vi "+S2C_M2p5942_Process.vi"(8 "Error In":errorcluster) -> (0 "Error Out":errorcluster)   [LabVIEW 2024]
uses:
  VIs/S2C_M2p5942_Proc_Globals.vi
panel:
  out "Err":bool
  in  "Clear":bool
  out "Exit":bool
  in  "LogDepth":u32=10 caption="Log Depth"
  in  "CtrlTab":T1(tab)
  in  "P1":T2={"Initialize"={"Index"=0, "IP Address"="<Not Used>", "Device"=0, "P1C1Exe"=FALSE}, "DeviceInfo"={"Device Name"="", "Serial Number"="", "Memory (MB)"="", "ClearExe"=FALSE}} {"Initialize"."Device" items=["Card", "digitizerNETBOX"]}
  in  "P2":T3={"Channels"={"CH1"={"CH0 Enable"=TRUE, "CH0 Range"=2, "CH0 Term"=0, "CH0 Type"=0, "CH0 Offset"=0}, "CH2"={"CH1 Enable"=TRUE, "CH1 Range"=2, "CH1 Term"=0, "CH1 Type"=0, "CH1 Offset"=0}, "CH3"={"CH2 Enable"=TRUE, "CH2 Range"=2, "CH2 Term"=0, "CH2 Type"=0, "CH2 Offset"=0}, "CH4"={"CH3 Enable"=TRUE, "CH3 Range"=2, "CH3 Term"=0, "CH3 Type"=0, "CH3 Offset"=0}, "P2C1Exe"=FALSE}, "Mode Settings"={"Mode"=0, "Memory"=16384, "Segment Size"=1024, "PostTrigger"=8192, "PreTrigger"=32, "ABA Mode"=16, "P2C2Exe"=FALSE}} {"Mode Settings"."ABA Mode" min=2 max=65535 step=1; "Mode Settings"."PostTrigger" min=4 step=4; "Mode Settings"."PreTrigger" min=4 max=8176 step=4; "Mode Settings"."Segment Size" min=8 step=4; "Mode Settings"."Memory" min=8 step=4; "Mode Settings"."Mode" items=["Singleshot", "Multiple Recording", "Gated Sampling", "ABA Mode"]; "Channels"."CH4"."CH3 Type" items=["Single-ended", "Differential"]; "Channels"."CH4"."CH3 Term" items=["1 MOhm", "50 Ohm"]; "Channels"."CH4"."CH3 Range" items=["±200 mV", "±500 mV", "±1000 mV", "±2000 mV", "±5000 mV", "±10000 mV"]; "Channels"."CH3"."CH2 Type" items=["Single-ended", "Differential"]; "Channels"."CH3"."CH2 Term" items=["1 MOhm", "50 Ohm"]; "Channels"."CH3"."CH2 Range" items=["±200 mV", "±500 mV", "±1000 mV", "±2000 mV", "±5000 mV", "±10000 mV"]; "Channels"."CH2"."CH1 Type" items=["Single-ended", "Differential"]; "Channels"."CH2"."CH1 Term" items=["1 MOhm", "50 Ohm"]; "Channels"."CH2"."CH1 Range" items=["±200 mV", "±500 mV", "±1000 mV", "±2000 mV", "±5000 mV", "±10000 mV"]; "Channels"."CH1"."CH0 Type" items=["Single-ended", "Differential"]; "Channels"."CH1"."CH0 Term" items=["1 MOhm", "50 Ohm"]; "Channels"."CH1"."CH0 Range" items=["±200 mV", "±500 mV", "±1000 mV", "±2000 mV", "±5000 mV", "±10000 mV"]}
  in  "P3":T4={"Trigger Settings"={"Trigger Source"=0, "External Trigger"=0, "EXT Trig Level 0"=1500, "EXT Trig Term"=TRUE, "Channel Trigger"=0, "CH Trig Level 0"=0, "CH Trig Level 1"=0, "Trigger Delay"=0, "P3C1Exe"=FALSE}, "Clock Settings"={"Clock Mode"=0, "Sampling Rate (kHz)"=10000.0, "Clock Output"=TRUE, "Termination"=TRUE, "Ref. Clock (MHz)"=10.0, "Threshold (mV)"=1500, "P3C2Exe"=FALSE}} {"Clock Settings"."Threshold (mV)" min=-5000 max=5000; "Clock Settings"."Sampling Rate (kHz)" min=1.0 max=5000000.0; "Clock Settings"."Ref. Clock (MHz)" min=0.0 max=125000.0; "Clock Settings"."Clock Mode" items=["Internal Clock Quartz", "External Clock", "External Reference Clock"]; "Trigger Settings"."Trigger Delay" max=65535 step=1; "Trigger Settings"."External Trigger" items=["None", "Pos. Edge", "Neg. Edge", "Any Edge", "High Level", "Low Level"]; "Trigger Settings"."Channel Trigger" items=["None", "Pos. Edge", "Neg. Edge", "Any Edge", "Pos. Rearm", "Neg. Rearm", "Enter Window", "Leave Window", "In Win", "Out Win"]; "Trigger Settings"."Trigger Source" items=["Software Trigger", "External Trigger", "Channel 0 Trigger", "Channel 1 Trigger", "Channel 2 Trigger", "Channel 3 Trigger", "Channel 4 Trigger", "Channel 5 Trigger", "Channel 6 Trigger", "Channel 7 Trigger"]}
  in  "P4":T5 {"Multi Purpose IO"."X3 Trigger Mode" items=["Pos. Edge", "Neg. Edge", "Any Edge", "High Level", "Low Level", "PW Long Pos.", "PW Long Neg.", "PW Short Pos.", "PW Short Neg."]; "Multi Purpose IO"."X2 Trigger Mode" items=["Pos. Edge", "Neg. Edge", "Any Edge", "High Level", "Low Level", "PW Long Pos.", "PW Long Neg.", "PW Short Pos.", "PW Short Neg."]; "Multi Purpose IO"."X1 Trigger Mode" items=["Pos. Edge", "Neg. Edge", "Any Edge", "High Level", "Low Level", "PW Long Pos.", "PW Long Neg.", "PW Short Pos.", "PW Short Neg."]; "Multi Purpose IO"."X3 Mode" items=["Disable", "Asynchronous Out", "Asynchronous In", "Trigger Out", "Trigger In", "Clock Out", "Digital In", "Show Run State", "Show Arm State", "Show Sync Arm State"]; "Multi Purpose IO"."X2 Mode" items=["Disable", "Asynchronous Out", "Asynchronous In", "Trigger Out", "Trigger In", "Clock Out", "Digital In", "Show Run State", "Show Arm State", "Show Sync Arm State"]; "Multi Purpose IO"."X1 Mode" items=["Disable", "Asynchronous Out", "Asynchronous In", "Trigger Out", "Trigger In", "Clock Out", "Digital In", "Show Run State", "Show Arm State", "Show Sync Arm State"]; "Multi Purpose IO"."X0 Mode" items=["Disable", "Asynchronous Out", "Trigger Out", "Clock Out", "Show Run State", "Show Arm State", "Show Sync Arm State"]}
  in  "P5":T6={"Acquisition"={"Single Shot"=FALSE, "Loop"=FALSE, "Force Trigger"=FALSE, "Status"="<Status>", "Stop"=FALSE, "Graph"=[]}}
  in  "CommLog":string caption="Communication Log"
  # "Main Cluster:\n394x886\n1 = 355x876\n2 = 355x438\n3 = 355x292\n4 = 163x438\n6 = 163x292\n8 = 163x219 \n\nSubTab 369x886\nSubClust 359x876"
  # "M2p5942 Driver Panel"
  # "Range"
  # "Term"
  # "Type"
  # "Offset"
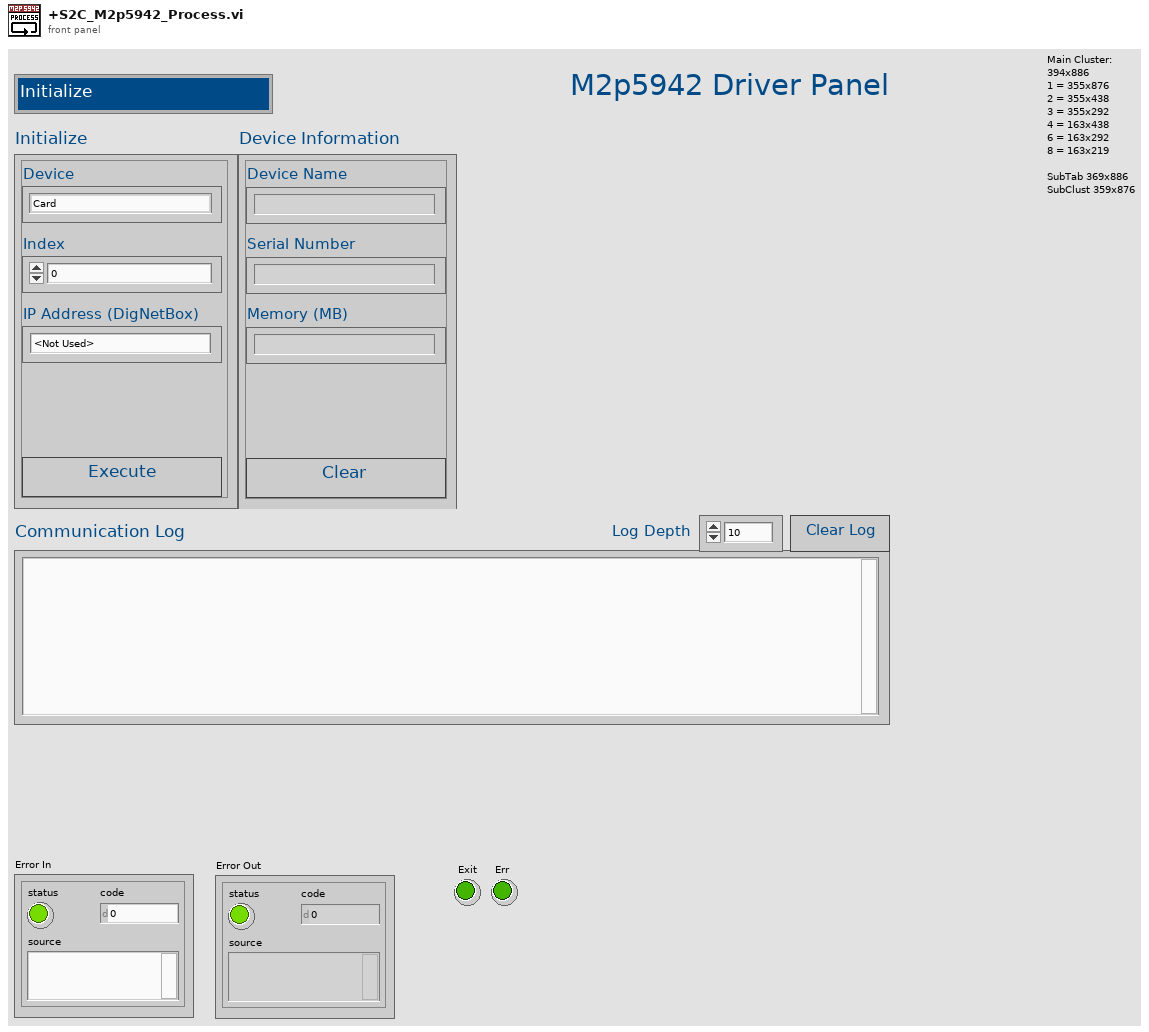
[diagram p1: front panel]
types:
  T1 = enum32{"Initialize", "Channels", "Trigger", "Multi Purpose IO", "Acquisition"}
  T2 = cluster{"Initialize":cluster{"Index":u32, "IP Address":string, "Device":u16, "P1C1Exe":bool}, "DeviceInfo":cluster{"Device Name":string, "Serial Number":string, "Memory (MB)":string, "ClearExe":bool}}
  T3 = cluster{"Channels":cluster{"CH1":cluster{"CH0 Enable":bool, "CH0 Range":u16, "CH0 Term":u16, "CH0 Type":u16, "CH0 Offset":i32}, "CH2":cluster{"CH1 Enable":bool, "CH1 Range":u16, "CH1 Term":u16, "CH1 Type":u16, "CH1 Offset":i32}, "CH3":cluster{"CH2 Enable":bool, "CH2 Range":u16, "CH2 Term":u16, "CH2 Type":u16, "CH2 Offset":i32}, "CH4":cluster{"CH3 Enable":bool, "CH3 Range":u16, "CH3 Term":u16, "CH3 Type":u16, "CH3 Offset":i32}, "P2C1Exe":bool}, "Mode Settings":cluster{"Mode":u16, "Memory":u32, "Segment Size":u32, "PostTrigger":u32, "PreTrigger":u32, "ABA Mode":u32, "P2C2Exe":bool}}
  T4 = cluster{"Trigger Settings":cluster{"Trigger Source":u16, "External Trigger":u16, "EXT Trig Level 0":i32, "EXT Trig Term":bool, "Channel Trigger":u16, "CH Trig Level 0":i32, "CH Trig Level 1":i32, "Trigger Delay":u32, "P3C1Exe":bool}, "Clock Settings":cluster{"Clock Mode":u16, "Sampling Rate (kHz)":dbl, "Clock Output":bool, "Termination":bool, "Ref. Clock (MHz)":dbl, "Threshold (mV)":i32, "P3C2Exe":bool}}
  T5 = cluster{"Multi Purpose IO":cluster{"X0 Mode":u16, "X1 Mode":u16, "X2 Mode":u16, "X3 Mode":u16, "X0 Send":bool, "X1 Send":bool, "X2 Send":bool, "X3 Send":bool, "X1 Trigger Mode":u16, "X2 Trigger Mode":u16, "X3 Trigger Mode":u16, "X1 Pulsewidth":u32, "X2 Pulsewidth":u32, "X3 Pulsewidth":u32, "ASync Read":bool, "ASync Data":i32}}
  T6 = cluster{"Acquisition":cluster{"Single Shot":bool, "Loop":bool, "Force Trigger":bool, "Status":string, "Stop":bool, "Graph":sgl[][]}}
  T7 = cluster{"Device Name":string, "Serial Number":string, "Memory (MB)":string, "ClearExe":bool}
  T8 = cluster{"Caller-Q":refnum<queue>, "Command":string, "Return":string, "Data":variant, "Timeout":dbl}
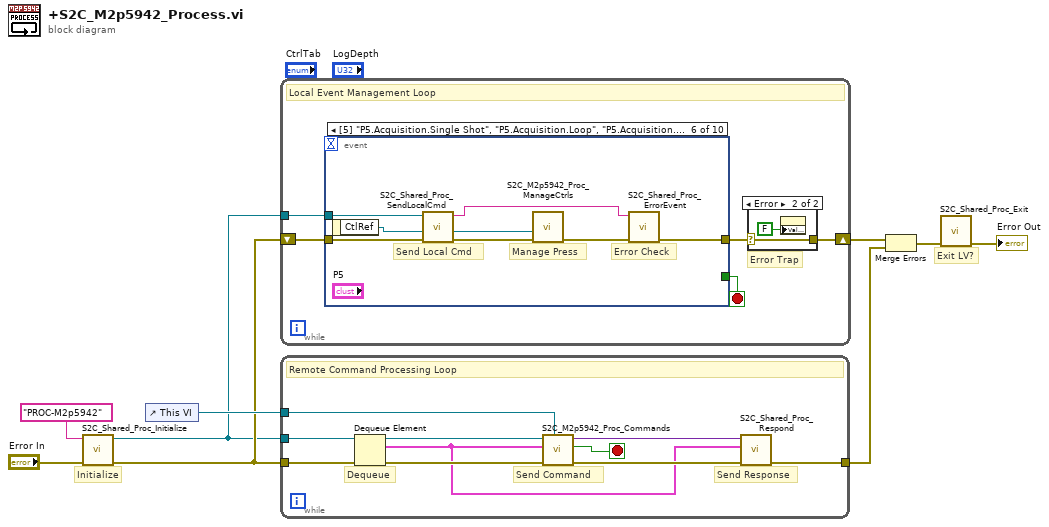
[diagram p0: block diagram]
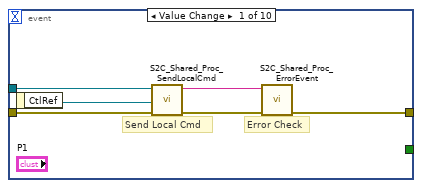
[diagram p3: hidden frame]
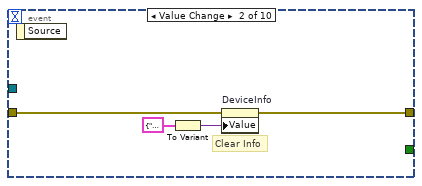
[diagram p4: hidden frame]
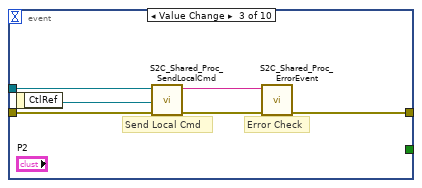
[diagram p5: hidden frame]
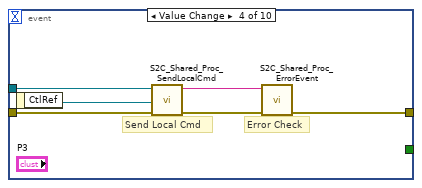
[diagram p6: hidden frame]
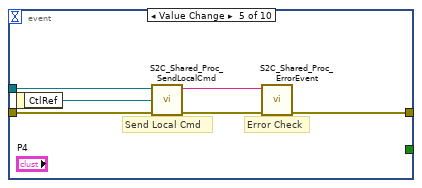
[diagram p7: hidden frame]
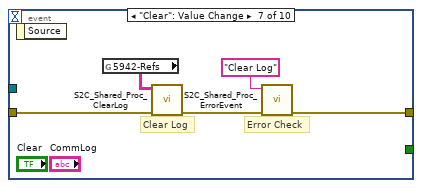
[diagram p8: hidden frame]
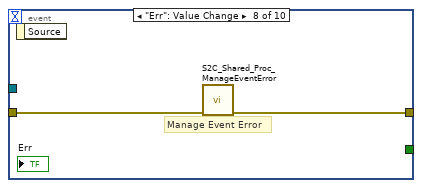
[diagram p9: hidden frame]
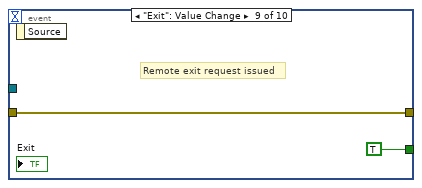
[diagram p10: hidden frame]
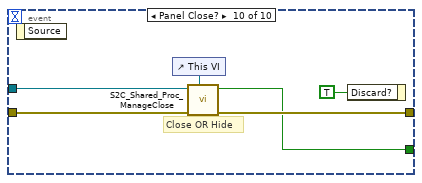
[diagram p11: hidden frame]
diagram:
  # "Exit LV?"
  # "Initialize"
  n1 = call "S2C_Shared_Proc_Initialize.vi"("Error In"="Error In", "Q-Name"="PROC-M2p5942" ("name (unnamed)")) -> ("Error Out"=w4:errorcluster, "Q-Ref"=w1:refnum<queue>)  [unwired: 8 in]
  n2 = control-ref of="This VI"() -> (w5:refnum<vi>)
  n3 = while {
    tunnel: w1 -> [w12]
    shift-right: [w10] -> w7
    shift-left: w4 -> [w14]
    stop <- w13 stop-if-true
    # "Error Trap"
    # "Local Event Management Loop"
    n4 = event shown="[5] \"P5.Acquisition.Single Shot\", \"P5.Acquisition.Loop\", \"P5.Acquisition.Stop\": Value Change" {
      selector: _ -> [_ _ _ _ _ _ _ _ _ _]
      dyn-events: _ -> [_ _ _ _ _ _ _ _ _ _]
      timeout: _ -> [_ _ _ _ _ _ _ _ _ _]
      tunnel: w14 -> [w23 w27 w33 w39 w43 w51 w57 w59 w61 w66]
      tunnel: w12 -> [w21 _ w31 w37 w41 w50 _ _ _ w64]
      tunnel: [w20 w26 w30 w36 w40 w49 w55 w58 w61 w65] -> w11
      tunnel: [_ _ _ _ _ _ _ _ TRUE ("Discard?") w63] -> w13
      event "P1.Initialize.P1C1Exe": Value Change {
        # "Error Check"
        # "Send Local Cmd"
        n5 = event-data() -> ("CtlRef"=w22:refnum<vi>)  [unwired: 1 in]
        n6 = call "S2C_Shared_Proc_SendLocalCmd.vi"("Error In"=w23, "ExeRef"=w22, "Q-Ref"=w21) -> ("Error Out"=w19:errorcluster, "Command"=w18:string)  [unwired: 7 in]
        n7 = call "S2C_Shared_Proc_ErrorEvent.vi"("Error In"=w19, "Command"=w18) -> ("Error Out"=w20:errorcluster)  [unwired: 9 in]
      }
      event "P1.DeviceInfo.ClearExe": Value Change {
        # "Clear Info"
        n8 = event-data() -> ()  [unwired: 1 in, 1 out]
        n9 = To Variant(anything=T7 {"Device Name"="", "Serial Number"="", "Memory (MB)"="", "ClearExe"=FALSE} ("DeviceInfo")) -> (Variant=w25:variant)
        n10 = property on="DeviceInfo" class="Clust"(error in=w27, "Value"=w25) -> (error out=w26:errorcluster)  [unwired: 1 in, 1 out]
      }
      event "P2.Channels.P2C1Exe", "P2.Mode Settings.P2C2Exe": Value Change {
        # "Error Check"
        # "Send Local Cmd"
        n11 = event-data() -> ("CtlRef"=w32:refnum<vi>)  [unwired: 1 in]
        n12 = call "S2C_Shared_Proc_SendLocalCmd.vi"("Error In"=w33, "ExeRef"=w32, "Q-Ref"=w31) -> ("Error Out"=w29:errorcluster, "Command"=w28:string)  [unwired: 7 in]
        n13 = call "S2C_Shared_Proc_ErrorEvent.vi"("Error In"=w29, "Command"=w28) -> ("Error Out"=w30:errorcluster)  [unwired: 9 in]
      }
      event "P3.Trigger Settings.P3C1Exe", "P3.Clock Settings.P3C2Exe": Value Change {
        # "Error Check"
        # "Send Local Cmd"
        n14 = event-data() -> ("CtlRef"=w38:refnum<vi>)  [unwired: 1 in]
        n15 = call "S2C_Shared_Proc_SendLocalCmd.vi"("Error In"=w39, "ExeRef"=w38, "Q-Ref"=w37) -> ("Error Out"=w35:errorcluster, "Command"=w34:string)  [unwired: 7 in]
        n16 = call "S2C_Shared_Proc_ErrorEvent.vi"("Error In"=w35, "Command"=w34) -> ("Error Out"=w36:errorcluster)  [unwired: 9 in]
      }
      event "P4.Multi Purpose IO.X0 Send", "P4.Multi Purpose IO.X1 Send", "P4.Multi Purpose IO.X2 Send", "P4.Multi Purpose IO.X3 Send", "P4.Multi Purpose IO.ASync Read": Value Change {
        # "Error Check"
        # "Send Local Cmd"
        n17 = event-data() -> ("CtlRef"=w42:refnum<vi>)  [unwired: 1 in]
        n18 = call "S2C_Shared_Proc_SendLocalCmd.vi"("Error In"=w43, "ExeRef"=w42, "Q-Ref"=w41) -> ("Error Out"=w45:errorcluster, "Command"=w44:string)  [unwired: 7 in]
        n19 = call "S2C_Shared_Proc_ErrorEvent.vi"("Error In"=w45, "Command"=w44) -> ("Error Out"=w40:errorcluster)  [unwired: 9 in]
      }
      event "P5.Acquisition.Single Shot", "P5.Acquisition.Loop", "P5.Acquisition.Stop": Value Change {
        # "Manage Press"
        # "Error Check"
        # "Send Local Cmd"
        n20 = event-data() -> ("CtlRef"=w46:refnum<vi>)  [unwired: 1 in]
        n21 = call "S2C_Shared_Proc_SendLocalCmd.vi"("Error In"=w51, "ExeRef"=w46, "Q-Ref"=w50) -> ("Error Out"=w48:errorcluster, "Command"=w52:string)  [unwired: 7 in]
        n22 = call "S2C_M2p5942_Proc_ManageCtrls.vi"("Error In"=w48, "CtlRef"=w46) -> ("Error Out"=w47:errorcluster)  [unwired: 9 in]
        n23 = call "S2C_Shared_Proc_ErrorEvent.vi"("Error In"=w47, "Command"=w52) -> ("Error Out"=w49:errorcluster)  [unwired: 9 in]
      }
      event "Clear": Value Change {
        # "Error Check"
        # "Clear Log"
        n24 = event-data() -> ()  [unwired: 1 in, 1 out]
        n25 = global read "S2C_M2p5942_Proc_Globals.vi" "5942-Refs"() -> (w53:string[][])
        n26 = call "S2C_Shared_Proc_ClearLog.vi"("Error In"=w57, "Refs"=w53) -> ("Error Out"=w56:errorcluster)  [unwired: 9 in]
        n27 = call "S2C_Shared_Proc_ErrorEvent.vi"("Error In"=w56, "Command"="Clear Log") -> ("Error Out"=w55:errorcluster)  [unwired: 9 in]
      }
      event "Err": Value Change {
        # "Manage Event Error"
        n28 = event-data() -> ()  [unwired: 1 in, 1 out]
        n29 = call "S2C_Shared_Proc_ManageEventError.vi"("Error In"=w59) -> ("Error Out"=w58:errorcluster)  [unwired: 10 in]
      }
      event "Exit": Value Change {
        # "Remote exit request issued"
        n30 = event-data() -> ()  [unwired: 1 in, 1 out]
      }
      event Panel Close? {
        # "Close OR Hide"
        n31 = event-data() -> ()  [unwired: 1 in, 1 out]
        n32 = control-ref of="This VI"() -> (w62:refnum<vi>)
        n33 = call "S2C_Shared_Proc_ManageClose.vi"("VI_Ref"=w62, "Error In"=w66, "Q-Ref"=w64) -> ("Error Out"=w65:errorcluster, "Exit?"=w63:bool)  [unwired: 7 in]
        n34 = event-data("Discard?"=TRUE) -> ()  [unwired: 1 in, 1 out]
      }
    }
    n35 = case shown="Error" w11 {
      selector: w11 -> [w15 w16]
      tunnel: [w15 w16] -> w10
      frame No Error {
      }
      frame Error {
        n36 = property on="Err" class="Bool (strict)"("Val(Sgnl)"=FALSE ("Value (Signaling)")) -> ()  [unwired: 2 in, 2 out]
      }
    }
  }
  n37 = while {
    tunnel: w1 -> [w70]
    tunnel: w5 -> [w72]
    tunnel: w4 -> [w77]
    tunnel: [w71] -> w6
    stop <- w73 stop-if-true
    # "Send Response"
    # "Send Command"
    # "Dequeue"
    # "Remote Command Processing Loop"
    n38 = Dequeue Element(queue=w70, error in (no error)=w77) -> (queue out=w69:refnum<queue>, element=w68:T8, error out=w76:errorcluster)  [unwired: 1 in, 1 out]
    n39 = call "S2C_M2p5942_Proc_Commands.vi"("VI_Ref"=w72, "Error In"=w76, "Settings"=w68, "Q-Ref"=w69) -> ("Error Out"=w74:errorcluster, "Stop?"=w73:bool, "Response"=w75:variant)  [unwired: 5 in]
    n40 = call "S2C_Shared_Proc_Respond.vi"("Error In"=w74, "Settings"=w68, "Response"=w75) -> ("Error Out"=w71:errorcluster)  [unwired: 8 in]
  }
  n41 = Merge Errors(w7, w6) -> (w3:errorcluster)
  n42 = call "S2C_Shared_Proc_Exit.vi"("Error In"=w3) -> ("Error Out"=→"Error Out":errorcluster)  [unwired: 10 in]
